vi "read slopes csv to cluster.vi"(8 "error in (no error)":errorcluster, 9 "Input Variables and Slopes in":T1 {"Feet of Stainless" format="%.2f"; "Height of Sample Box" format="%.2f"; "Reservoir Pressure" format="%.2f"; "Flow Offset" format="%.2f"; "String Pot Offset" format="%.2f"; "Aux 3 Offset" format="%.2f"; "Aux 2 Offset" format="%.2f"; "Aux 1 Offset" format="%.2f"; "Aux 3 Slope" format="%.2f"; "Aux 2 Slope" format="%.2f"; "Aux 1 Slope" format="%.2f"; "Up Hole  Pressure Offset" format="%.2f"; "DH Pressure Offset" format="%.2f"; "DH Pressure Trans Slope" format="%.2f"; "Atmospheric Pressure" format="%.2f"; "Depth to Water Table" format="%.2f"; "Up Hole Pressure Slope" format="%.2f"; "Flow Slope" format="%.2f"; "String Pot Slope" format="%.2f"; "Total Volume" format="%.2f"}, 10 "Slopes File Path":path, 11 "Data Setup Indicator in":refnum<vi>) -> (0 "error out":errorcluster, 3 "Input Variables and Slopes out":T1 {"Feet of Stainless" format="%.2f"; "Height of Sample Box" format="%.2f"; "Reservoir Pressure" format="%.2f"; "Flow Offset" format="%.2f"; "String Pot Offset" format="%.2f"; "Aux 3 Offset" format="%.2f"; "Aux 2 Offset" format="%.2f"; "Aux 1 Offset" format="%.2f"; "Aux 3 Slope" format="%.2f"; "Aux 2 Slope" format="%.2f"; "Aux 1 Slope" format="%.2f"; "Up Hole  Pressure Offset" format="%.2f"; "DH Pressure Offset" format="%.2f"; "DH Pressure Trans Slope" format="%.2f"; "Atmospheric Pressure" format="%.2f"; "Depth to Water Table" format="%.2f"; "Up Hole Pressure Slope" format="%.2f"; "Flow Slope" format="%.2f"; "String Pot Slope" format="%.2f"; "Total Volume" format="%.2f"})   [LabVIEW 2016]
uses:
  KPRO_2016 subvis/Control 2.ctl
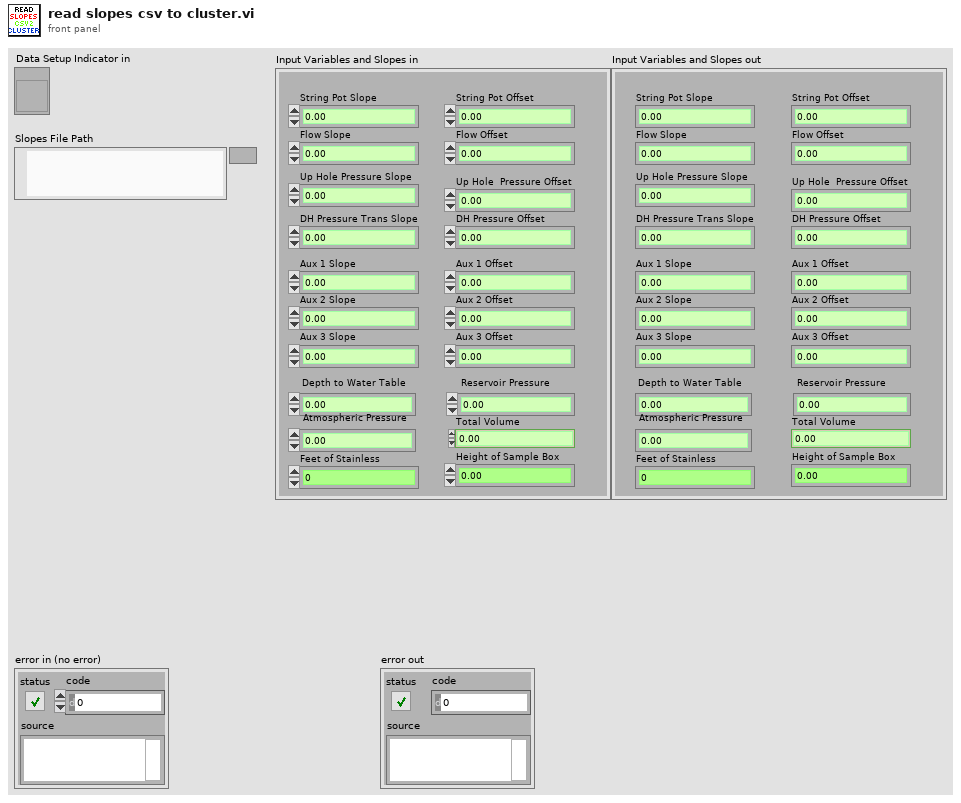
[diagram p1: front panel]
types:
  T1 = typedef "Control 2.ctl" = cluster{"Total Volume":dbl, "String Pot Slope":dbl, "Flow Slope":dbl, "Up Hole Pressure Slope":dbl, "Depth to Water Table":dbl, "Atmospheric Pressure":dbl, "DH Pressure Trans Slope":dbl, "DH Pressure Offset":dbl, "Up Hole  Pressure Offset":dbl, "Aux 1 Slope":dbl, "Aux 2 Slope":dbl, "Aux 3 Slope":dbl, "Aux 1 Offset":dbl, "Aux 2 Offset":dbl, "Aux 3 Offset":dbl, "String Pot Offset":dbl, "Flow Offset":dbl, "Reservoir Pressure":dbl, "Height of Sample Box":dbl, "Feet of Stainless ":i32}
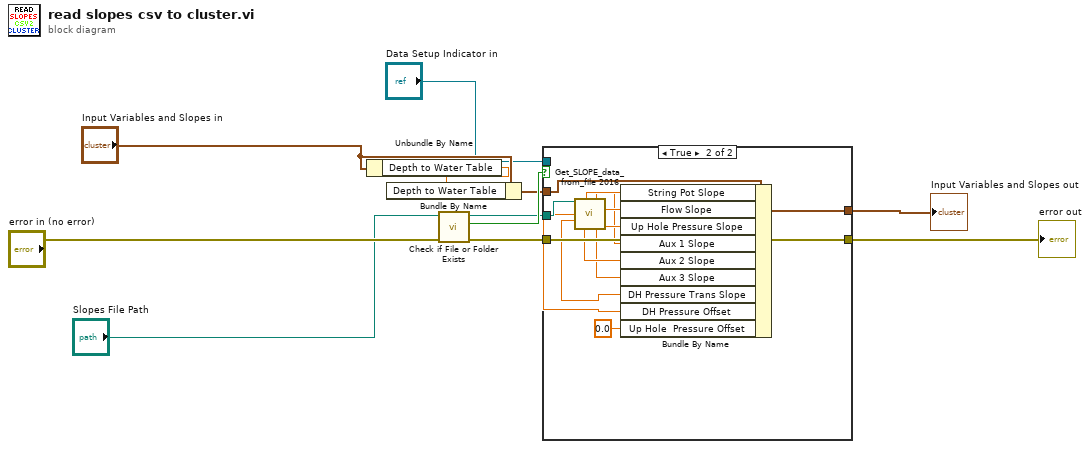
[diagram p0: block diagram]
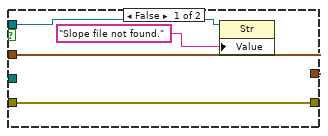
[diagram p2: hidden frame]
diagram:
  n1 = Unbundle By Name("Input Variables and Slopes in") -> ("Depth to Water Table"=w3:dbl)
  n2 = Bundle By Name(cluster="Input Variables and Slopes in", "Depth to Water Table"=w3) -> (w6:T1)
  n3 = call <vilib>:"Check if File or Folder Exists.vi"("error in (no error)"="error in (no error)", "path"="Slopes File Path") -> ("error out"=w9:errorcluster, "file or folder exists?"=w10:bool, "dup path"=w5:path)  [unwired: 7 in]
  n4 = case shown="True" w10 {
    tunnel: w5 -> [_ w28]
    tunnel: w6 -> [w15 w27]
    tunnel: [w15 w26] -> w7
    tunnel: w9 -> [w14 w22]
    tunnel: [w14 w22] -> w8
    tunnel: "Data Setup Indicator in" -> [w12 _]
    frame False {
      n5 = property class="Str"(reference=w12, "Value"="Slope file not found." ("Data Setup Indicator")) -> ()  [unwired: 1 in, 2 out]
    }
    frame True {
      n6 = call "Get_SLOPE_data_from_file 2016.vi"("Slopes File Path"=w28) -> ("Last Aux 1 Slope"=w21:dbl, "Last_String_Pot_Slope"=w25:dbl, "DHT Offset"=w17:dbl, "DHT Slope"=w18:dbl, "Last_Flow_Slope"=w24:dbl, "Last Aux 2 Slope"=w20:dbl, "Last Aux 3 Slope"=w19:dbl, "Last_Pressure_Slope"=w23:dbl)  [unwired: 5 in, 2 out]
      n7 = Bundle By Name(cluster=w27, "String Pot Slope"=w25, "Flow Slope"=w24, "Up Hole Pressure Slope"=w23, "Aux 1 Slope"=w21, "Aux 2 Slope"=w20, "Aux 3 Slope"=w19, "DH Pressure Trans Slope"=w18, "DH Pressure Offset"=w17, "Up Hole  Pressure Offset"=0.0) -> (w26:T1)
    }
  }
  "error out" <- w8
  "Input Variables and Slopes out" <- w7
